vi "mouse_ctrl set_move_pos.vi"(8 "error in (no error)":errorcluster, 10 "xy pos":cluster{"X":dbl, "Y":dbl}, 11 "mouse_ctrl in":refnum<class "mouse_ctrl.lvclass">) -> (0 "error out":errorcluster, 3 "mouse_ctrl out":refnum<class "mouse_ctrl.lvclass">)   [LabVIEW 2018, in "mouse_ctrl.lvclass"]
uses:
  mouse_ctrl.lvclass
  mouse_ctrl.lvclass/mouse_ctrl.ctl
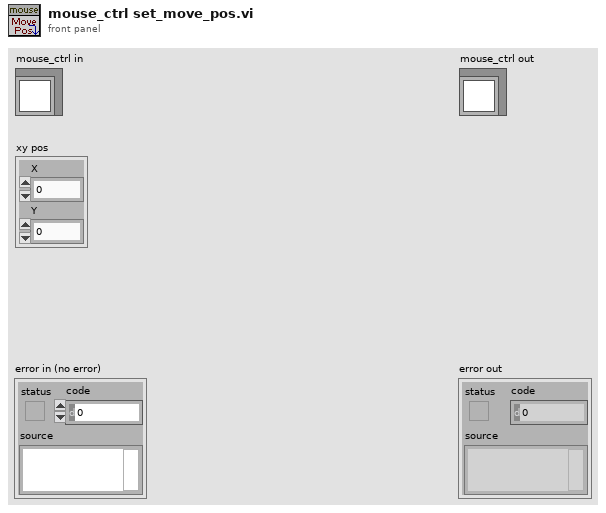
[diagram p1: front panel]
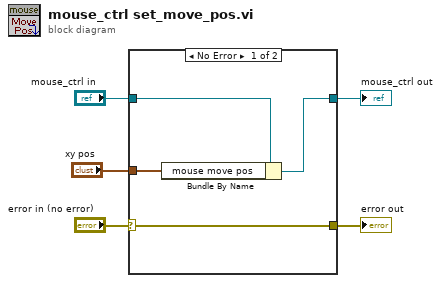
[diagram p0: block diagram]
diagram:
  n1 = case shown="No Error" "error in (no error)" {
    selector: "error in (no error)" -> [w9 w11]
    tunnel: [w9 w11] -> w3
    tunnel: [w8 w10] -> w2
    tunnel: "mouse_ctrl in" -> [w7 w10]
    tunnel: "xy pos" -> [w6 _]
    frame No Error {
      n2 = Bundle By Name(cluster=w7, "mouse move pos"=w6) -> (w8:refnum<class "mouse_ctrl.lvclass">)
    }
    frame Error {
    }
  }
  "error out" <- w3
  "mouse_ctrl out" <- w2
